vi "AddCoordinate.vi"(8 "error in (no error)":errorcluster, 11 "Snake in":refnum<class "Snake.lvclass">) -> (0 "error out":errorcluster, 3 "Snake out":refnum<class "Snake.lvclass">)   [LabVIEW 2019, in "RT_Game.lvlib" / "Snake.lvclass"]
uses:
  Snake.lvclass
  Snake.lvclass/Snake.ctl
  SnakeGame/CoordinateData.ctl
  Game/Coordinate.ctl
  Game/Game.lvclass
  SnakeGame/SnakeGame.lvclass
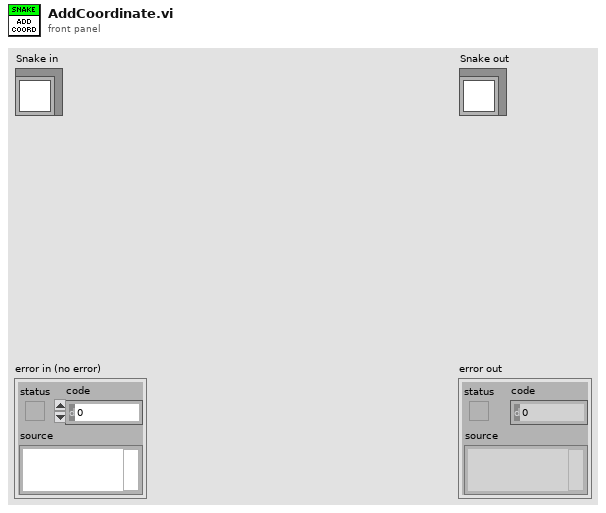
[diagram p1: front panel]
types:
  T1 = typedef "RT_Game.lvlib/SnakeGame.lvclass/CoordinateData.ctl" = cluster{"Coordinate":T2, "TileCode":u32}
  T2 = typedef "RT_Game.lvlib/Game.lvclass/Coordinate.ctl" = cluster{"x":dbl, "y":dbl}
  T3 = typedef "RT_Game.lvlib/SnakeGame.lvclass/Direction.ctl" = enum16{"Up", "Left", "Down", "Right"}
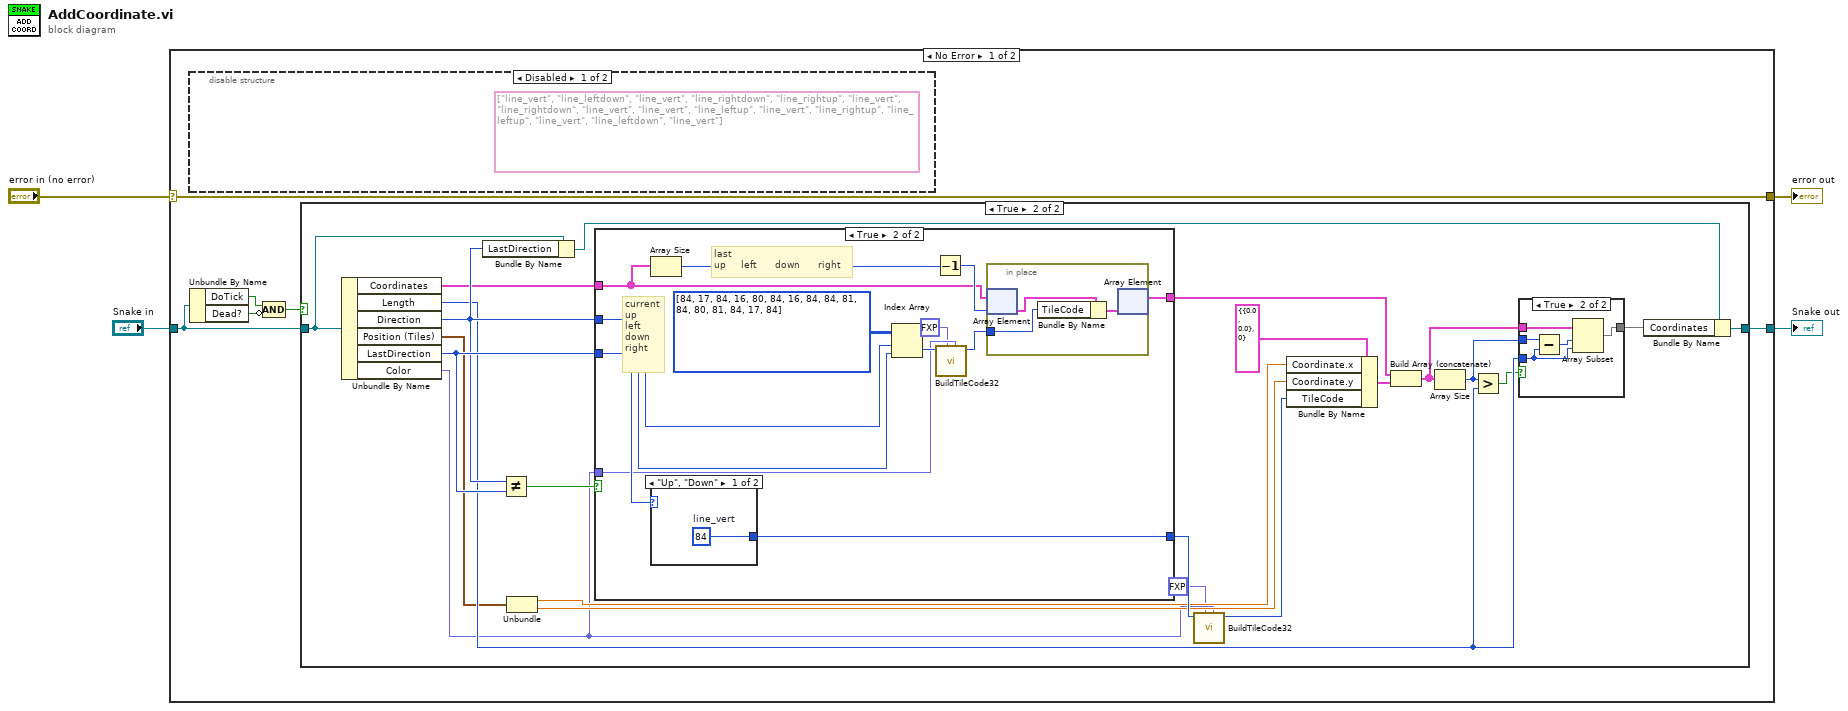
[diagram p0: block diagram]
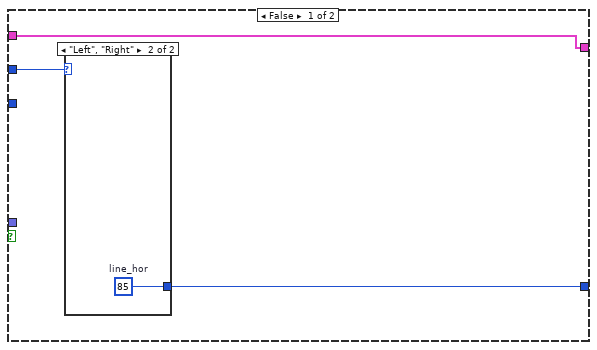
[diagram p3: hidden frame]
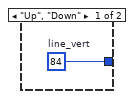
[diagram p4: hidden frame]
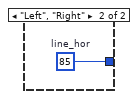
[diagram p5: hidden frame]
diagram:
  n1 = case shown="No Error" "error in (no error)" {
    selector: "error in (no error)" -> [w10 w63]
    tunnel: [w10 w63] -> w3
    tunnel: [w9 w62] -> w1
    tunnel: "Snake in" -> [w8 w62]
    frame No Error {
      n2 = disable-structure shown="Disabled" {
        frame Disabled {
          (unwired) string[][] [["line_vert", "line_leftdown", "line_vert", "line_rightdown"], ["line_rightup", "line_vert", "line_rightdown", "line_vert"], ["line_vert", "line_leftup", "line_vert", "line_rightup"], ["line_leftup", "line_vert", "line_leftdown", "line_vert"]] ("Array")
        }
        frame Enabled {
        }
      }
      n3 = Unbundle By Name(w8) -> ("DoTick"=w5:bool, "Dead?"=w7:bool)
      n4 = Compound Arithmetic op=AND(w5, invert w7) -> (w6:bool)
      n5 = case shown="True" w6 {
        tunnel: w8 -> [w11 w15]
        tunnel: [w11 w14] -> w9
        frame False {
        }
        frame True {
          n6 = Unbundle By Name(w15) -> ("Coordinates"=w25:T1[], "Length"=w27:i16, "Direction"=w30:T3, "Position (Tiles)"=w26:T2, "LastDirection"=w31:T3, "Color"=w13:fxp<+,3,3>)
          n7 = Bundle By Name(cluster=w15, "LastDirection"=w30) -> (w29:refnum<class "Snake.lvclass">)
          n8 = Not Equal?(x=w30, y=w31) -> (x != y?=w19:bool)
          n9 = Unbundle(w26) -> ("x"=w17:dbl, "y"=w16:dbl)
          n10 = case shown="True" w19 {
            tunnel: w30 -> [w36 w45]
            tunnel: w31 -> [_ w50]
            tunnel: [w35 w44] -> w33
            tunnel: w25 -> [w34 w47]
            tunnel: [w34 w46] -> w18
            tunnel: w13 -> [_ w40]
            frame False {
              n11 = case shown="\"Left\", \"Right\"" w36 {
                tunnel: [w37 w38] -> w35
                frame "Up", "Down" {
                  w37 = u16 84  # line_vert
                }
                frame "Left", "Right" {
                  w38 = u16 85  # line_hor
                }
              }
            }
            frame True {
              # "last\nup     left      down      right"
              # "current\nup\nleft\ndown\nright"
              n12 = Array Size(array=w47) -> (size(s)=w49:i32)
              n13 = case shown="\"Up\", \"Down\"" w45 {
                tunnel: [w51 w52] -> w44
                frame "Up", "Down" {
                  w51 = u16 84  # line_vert
                }
                frame "Left", "Right" {
                  w52 = u16 85  # line_hor
                }
              }
              n14 = Index Array(array=u16[][] [[84, 17, 84, 16], [80, 84, 16, 84], [84, 81, 84, 80], [81, 84, 17, 84]] ("Array"), index (row)=w45, index (col)=w50) -> (element=w43:u16)
              n15 = Decrement(x=w49) -> (x-1=w48:i32)
              n16 = call "BuildTileCode32.vi"("replacecolor"=w40, "color_to_replace"=fxp<+,3,3> 7.0, "Tilenumber"=w43) -> ("TileCode"=w42:u32)  [unwired: 8 in]
              n17 = in-place {
                in-place-border: w42 -> [w53]
                n18 = in-place-array #1(w47, w48) -> (w55:T1)
                n19 = Bundle By Name(cluster=w55, "TileCode"=w53) -> (w54:T1)
                n20 = in-place-array #1(w54) -> (w46:T1[])  [unwired: 1 out]
              }
            }
          }
          n21 = call "BuildTileCode32.vi"("replacecolor"=w13, "color_to_replace"=fxp<+,3,3> 7.0, "Tilenumber"=w33) -> ("TileCode"=w32:u32)  [unwired: 8 in]
          n22 = Bundle By Name(cluster=T1 {"Coordinate"={"x"=0.0, "y"=0.0}, "TileCode"=0} ("Coordinate"), "Coordinate.x"=w17, "Coordinate.y"=w16, "TileCode"=w32) -> (w20:T1)
          n23 = Build Array (concatenate)(w18, w20) -> (w22:T1[])
          n24 = Array Size(array=w22) -> (size(s)=w23:i32)
          n25 = Greater?(x=w23, y=w27) -> (0:w24:bool)
          n26 = case shown="True" w24 {
            tunnel: [w56 w61] -> w28
            tunnel: w22 -> [w56 w60]
            tunnel: w23 -> [_ w59]
            tunnel: w27 -> [_ w57]
            frame False {
            }
            frame True {
              n27 = Subtract(x=w59, y=w57) -> (x-y=w58:i32)
              n28 = Array Subset(array=w60, index=w58, length=w57) -> (w61:T1[])
            }
          }
          n29 = Bundle By Name(cluster=w29, "Coordinates"=w28) -> (w14:refnum<class "Snake.lvclass">)
        }
      }
    }
    frame Error {
    }
  }
  "error out" <- w3
  "Snake out" <- w1
